vi "Control.vi"(8 "error in (no error)":errorcluster, 10 "command (show)":T1=1 items=["show"=1, "hide"=2, "exit"=3]) -> (0 "error out":errorcluster, 2 "return value":i32)   [LabVIEW 2017, in "HighFinesse WS5.lvlib"]
doc: "Show, hides, or exits the wavelength meter (WLM) server. If the server is not running, and either show or hide are called, it will start."
uses:
  HighFinesse WS5.lvlib
  Control typedefs.llb/Control Action.ctl
  <vilib>/Utility/error.llb/DialogType.ctl
  wlmData.dll
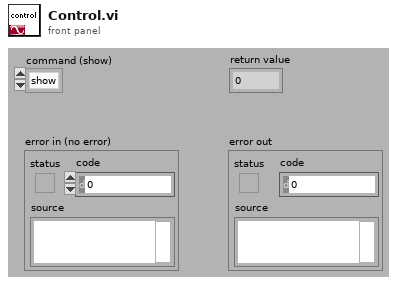
[diagram p1: front panel]
types:
  T1 = typedef "Control Action.ctl" = u32
  T2 = typedef "DialogType.ctl" = u16
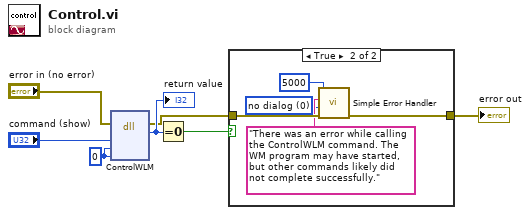
[diagram p0: block diagram]
diagram:
  w7 = 0 ("Res1")
  n1 = dll-call lib="C:/LabVIEW-programs-dev/Instruments/Wavelength meter/HighFinesse WS5/wlmData.dll" fn="ControlWLM"(error in="error in (no error)", "Action"="command (show)", "App"=w7, "Res1"=w7) -> (error out=w4:errorcluster, "return type"=w6:i32)  [unwired: 5 in, 1 out]
  "return value" <- w6
  n2 = Equal To 0?(x=w6) -> (x = 0?=w5:bool)
  n3 = case shown="True" w5 {
    tunnel: w4 -> [w8 w13]
    tunnel: [w8 w10] -> w2
    frame False {
    }
    frame True {
      w11 = T2 0 items=["no dialog", "OK message", "continue or stop message", "OK message + warnings", "continue/stop + warnings"] ("type of dialog (OK msg:1)")
      n4 = call <vilib>:"Simple Error Handler.vi"("error code (no error:0)"=5000, "error source (\" \")"="There was an error while calling the ControlWLM command. The WM program may have started, but other commands likely did not complete successfully." ("error source (\" \")"), "type of dialog (OK msg:1)"=w11, "error in (no error)"=w13) -> ("error out"=w10:errorcluster)  [unwired: 5 out]
    }
  }
  "error out" <- w2
